vi "ConvertAbsolutePathToRelative.vi"(11 "Absolute Path":path) -> (3 "Relative Path":path)   [LabVIEW 2018]
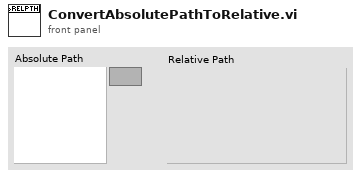
[diagram p1: front panel]
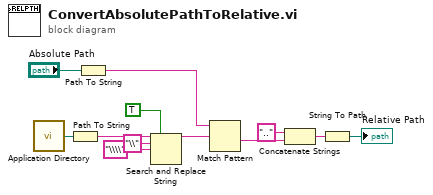
[diagram p0: block diagram]
diagram:
  n1 = call <vilib>:"Application Directory.vi"() -> ("Application Directory"=w10:path)
  n2 = Path To String(path=w10) -> (string=w7:string)
  n3 = Path To String(path="Absolute Path") -> (string=w11:string)
  n4 = Search and Replace String(replace all?=TRUE ("replace all? (F)"), input string=w7, search string="\\", replace string="\\\\" ("replace string (\"\")")) -> (result string=w6:string)  [unwired: 4 in, 3 out]
  n5 = Match Pattern(string=w11, regular expression=w6) -> (after substring=w12:string)  [unwired: 1 in, 3 out]
  n6 = Concatenate Strings(".." ("string"), w12) -> (w2:string)
  n7 = String To Path(string=w2) -> (path=→"Relative Path":path)
